vi "Read XBox Controller Layout.vi"(8 "error in (no error)":errorcluster, 11 "XBoxController in":refnum<class "XBoxController.lvclass">) -> (0 "error out":errorcluster, 2 "XBox Controller Layout":T1 {"Right Joystick Right" scale=-1.0..1.0; "Left Joystick Right" scale=-1.0..1.0; "Right Joystick Forward" scale=-1.0..1.0; "Left Joystick Forward" scale=-1.0..1.0}, 3 "XBoxController out":refnum<class "XBoxController.lvclass">)   [LabVIEW 2013, in "XBoxController.lvclass"]
uses:
  XBoxController.lvclass
  XBoxController.lvclass/XBoxController.ctl
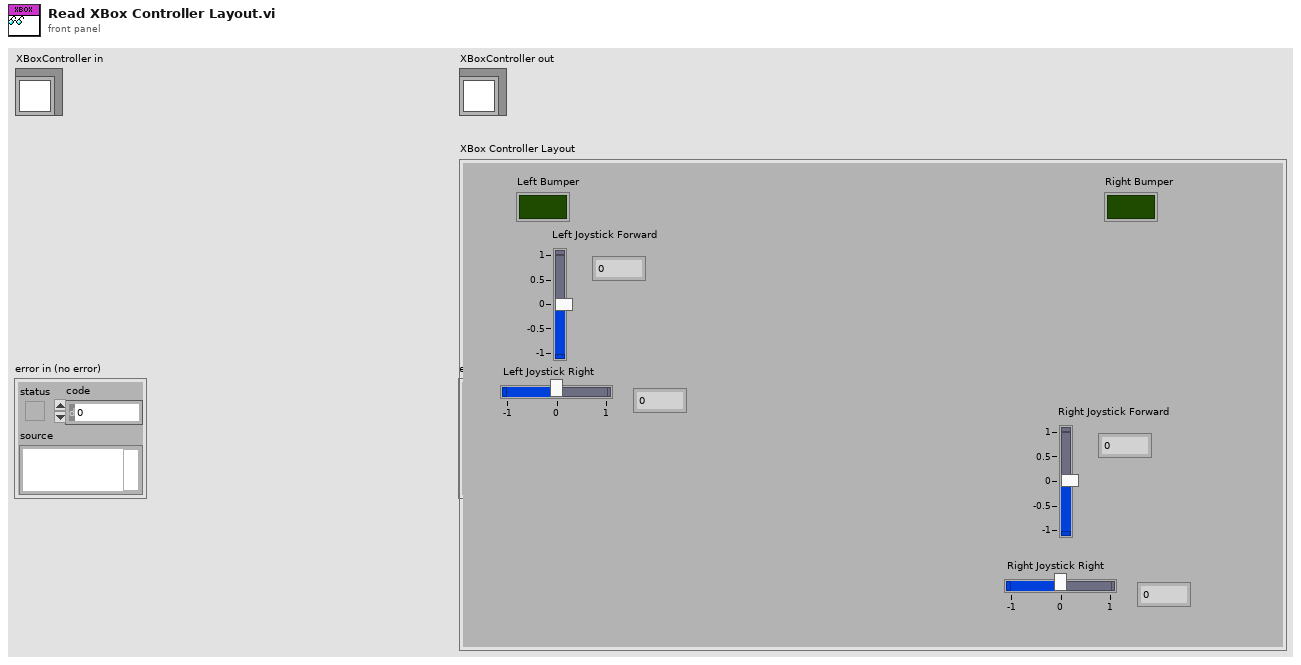
[diagram p1: front panel]
types:
  T1 = cluster{"Left Bumper":bool, "Right Bumper":bool, "Left Joystick Forward":dbl, "Left Joystick Right":dbl, "Right Joystick Forward":dbl, "Right Joystick Right":dbl}
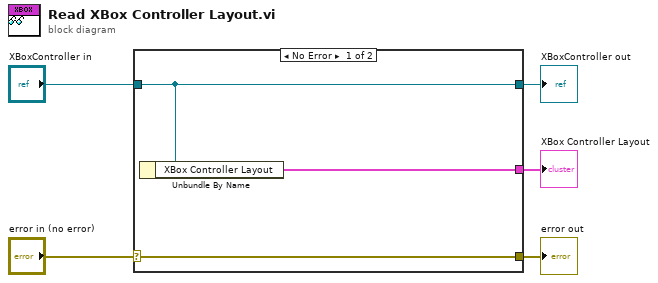
[diagram p0: block diagram]
diagram:
  n1 = case shown="No Error" "error in (no error)" {
    selector: "error in (no error)" -> [w8 w9]
    tunnel: [w8 w9] -> w4
    tunnel: [w7 w10] -> w2
    tunnel: "XBoxController in" -> [w7 w10]
    tunnel: [w6 _] -> w1
    frame No Error {
      n2 = Unbundle By Name(w7) -> ("XBox Controller Layout"=w6:T1)
    }
    frame Error {
    }
  }
  "error out" <- w4
  "XBoxController out" <- w2
  "XBox Controller Layout" <- w1
